vi "FT10_Config Bundle Analysis.vi"(8 "error in (no error)":errorcluster, 10 "Config String Value Cluster":T1) -> (0 "error out":errorcluster, 2 "Config cluster":T5={"Unitherm Port"="COM4", "Simulate Values"=TRUE, "Fornax Connect Attempts"=0})   [LabVIEW 2015]
doc: "Analyze key values and convert to correct data type"
uses:
  Controls/Control_Config Cluster.ctl
  Controls/Control_Config Unitherm Port.ctl
  Controls/Control_Config Simulate Values.ctl
  Controls/Control_Config Fornax Connect Attempts.ctl
  Controls/Control_Config Str Val Cluster.ctl
  Controls/Control_Config Unitherm Str Val.ctl
  Controls/Control_Config Simulation Str Val.ctl
  Controls/Control_Config Fornax Attempts Str Val.ctl
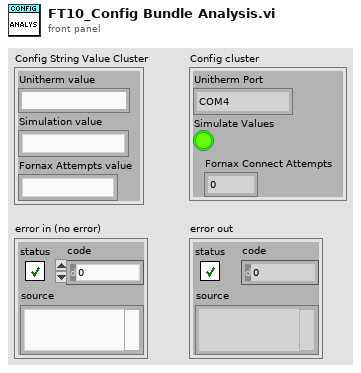
[diagram p1: front panel]
types:
  T1 = typedef "Control_Config Str Val Cluster.ctl" = cluster{"Unitherm value":T2, "Simulation value":T3, "Fornax Attempts value":T4}
  T2 = typedef "Control_Config Unitherm Str Val.ctl" = string
  T3 = typedef "Control_Config Simulation Str Val.ctl" = string
  T4 = typedef "Control_Config Fornax Attempts Str Val.ctl" = string
  T5 = typedef "Control_Config Cluster.ctl" = cluster{"Unitherm Port":T6, "Simulate Values":T7, "Fornax Connect Attempts":T8}
  T6 = typedef "Control_Config Unitherm Port.ctl" = string
  T7 = typedef "Control_Config Simulate Values.ctl" = bool
  T8 = typedef "Control_Config Fornax Connect Attempts.ctl" = i32
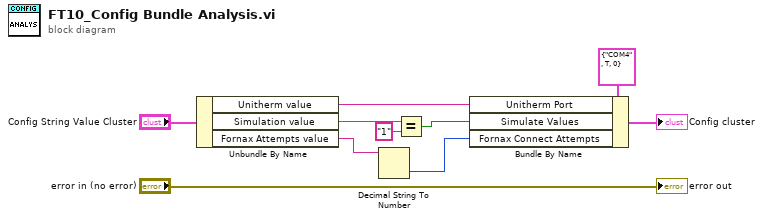
[diagram p0: block diagram]
diagram:
  n1 = Unbundle By Name("Config String Value Cluster") -> ("Unitherm value"=w7:T2, "Simulation value"=w8:T3, "Fornax Attempts value"=w9:T4)
  n2 = Decimal String To Number(string=w9) -> (number=w5:i32)  [unwired: 2 in, 1 out]
  n3 = Equal?(x=w8, y="1") -> (x = y?=w2:bool)
  n4 = Bundle By Name(cluster=T5 {"Unitherm Port"="COM4", "Simulate Values"=TRUE, "Fornax Connect Attempts"=0}, "Unitherm Port"=w7, "Simulate Values"=w2, "Fornax Connect Attempts"=w5) -> (→"Config cluster":T5)
  "error out" <- "error in (no error)"
